vi "Get Date Time String.vi"() -> (3 "Time String":string)   [LabVIEW 2020, in "ProjectBuilder.lvlib"]
uses:
  ProjectBuilder.lvlib
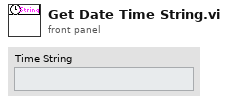
[diagram p1: front panel]
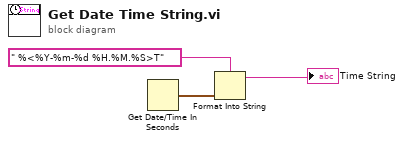
[diagram p0: block diagram]
diagram:
  n1 = Get Date/Time In Seconds() -> (seconds since 1Jan1904=w1:timestamp)
  n2 = Format Into String(format string=" %<%Y-%m-%d %H.%M.%S>T" ("initial string"), w1) -> (resulting string=→"Time String":string)  [unwired: 2 in, 1 out]
